vi "SetFormat.vi"(1 "NPframetransfer":i32=512, 3 "NStotal":i32=512, 4 "NSdark":i32, 5 "NPoverscan":i32, 6 "NPunderscan":i32, 7 "NPdark":i32, 8 "NSunderscan":i32, 9 "NPtotal":i32=512, 10 "NSoverscan":i32) -> (2 "Error":bool)   [LabVIEW 2014]
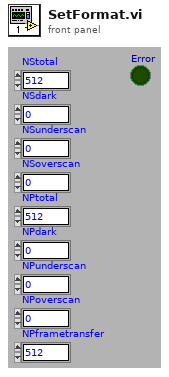
[diagram p1: front panel]
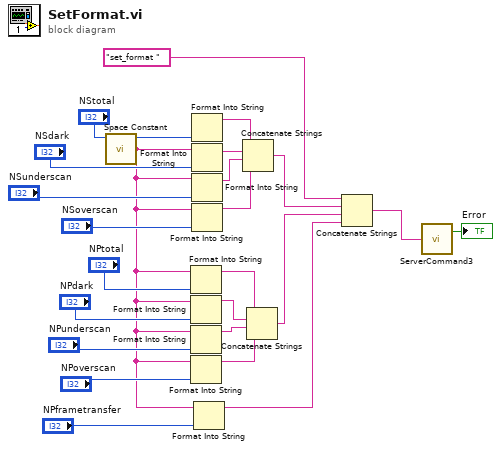
[diagram p0: block diagram]
diagram:
  n1 = call <vilib>:"Space Constant.vi"() -> ("String"=w2:string)
  n2 = Format Into String(initial string=w2, "NPtotal") -> (resulting string=w12:string)  [unwired: 2 in, 1 out]
  n3 = Format Into String(initial string=w2, "NPdark") -> (resulting string=w11:string)  [unwired: 2 in, 1 out]
  n4 = Format Into String(initial string=w2, "NPunderscan") -> (resulting string=w10:string)  [unwired: 2 in, 1 out]
  n5 = Format Into String(initial string=w2, "NPoverscan") -> (resulting string=w9:string)  [unwired: 2 in, 1 out]
  n6 = Format Into String("NStotal") -> (resulting string=w23:string)  [unwired: 3 in, 1 out]
  n7 = Format Into String(initial string=w2, "NSdark") -> (resulting string=w22:string)  [unwired: 2 in, 1 out]
  n8 = Format Into String(initial string=w2, "NSunderscan") -> (resulting string=w21:string)  [unwired: 2 in, 1 out]
  n9 = Format Into String(initial string=w2, "NSoverscan") -> (resulting string=w8:string)  [unwired: 2 in, 1 out]
  n10 = Format Into String(initial string=w2, "NPframetransfer") -> (resulting string=w3:string)  [unwired: 2 in, 1 out]
  n11 = Concatenate Strings(w23, w22, w21, w8) -> (w5:string)
  n12 = Concatenate Strings(w12, w11, w10, w9) -> (w4:string)
  n13 = Concatenate Strings("set_format " ("Command"), w5, w4, w3) -> (w6:string)
  n14 = call "ServerCommand3.vi"("Command"=w6) -> ("Error"=→"Error":bool)  [unwired: 1 out]
